vi "Do.vi"(8 "error in (no error)":errorcluster, 10 "Actor in":refnum<class "Actor.lvclass">, 11 "Initiate Acquisition Msg":refnum<class "Initiate Acquisition Msg.lvclass">) -> (0 "error out":errorcluster, 2 "Actor out":refnum<class "Actor.lvclass">)   [LabVIEW 2015, in "CS++Scope.lvlib" / "Initiate Acquisition Msg.lvclass"]
doc: "This VI delivers the message to the actor by calling the appropriate method(s) on the actor."
uses:
  Initiate Acquisition Msg.lvclass
  CS++Scope/CS++Scope.lvclass
  CSPP_Core/Actors/CS++PVMonitor Messages/CS++PVUpdate Msg/CS++PVUpdate Msg.lvclass
  CSPP_Core/Classes/CS++ProcessVariables/ProcessVariable/PV.lvclass
  <vilib>/ActorFramework/Actor/Actor.lvclass
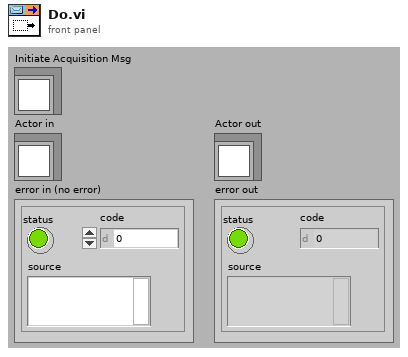
[diagram p1: front panel]
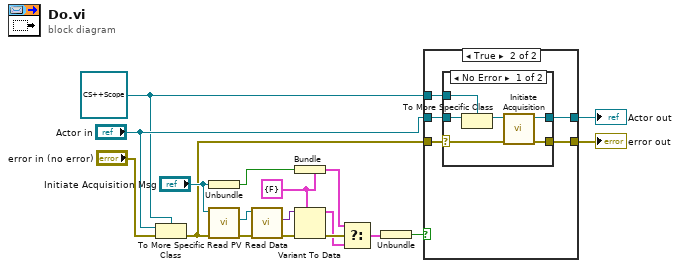
[diagram p0: block diagram]
diagram:
  w4 = cluster{bool} {FALSE} ("Type")
  w14 = refnum<class "CS++Scope.lvclass"> refnum ("Actor in")
  n1 = To More Specific Class(target class=w14, reference="Actor in", error in="error in (no error)") -> (error out=w12:errorcluster)  [unwired: 1 out]
  n2 = Unbundle ("Pre-Unbundler")("Initiate Acquisition Msg") -> (w1:bool)
  n3 = call "Read PV.vi"("error in (no error)"=w12, "CS++PVUpdate Msg in"="Initiate Acquisition Msg") -> ("error out"=w11:errorcluster, "PV"=w3:refnum<class "PV.lvclass">)  [unwired: 7 in, 1 out]
  n4 = call "Read Data.vi"("error in (no error)"=w11, "PV in"=w3) -> ("error out"=w9:errorcluster, "Data"=w10:variant)  [unwired: 7 in, 1 out]
  n5 = Bundle ("Pre-Bundler")(cluster=w4, w1) -> (w7:cluster{bool})
  n6 = Variant To Data(error in=w9, type=w4, Variant=w10) -> (data=w6:cluster{bool}, error out=w8:errorcluster)
  n7 = Select(t=w7, s=w8, f=w6) -> (s? t:f=w5:cluster{bool})
  n8 = Unbundle ("Main-Unbundler")(w5) -> (w2:bool)
  n9 = case "Execute?" shown="True" w2 {
    tunnel: [w19 w25] -> w17
    tunnel: [w20 w24] -> w16
    tunnel: "Actor in" -> [w20 w23]
    tunnel: w14 -> [_ w22]
    tunnel: w12 -> [w19 w21]
    frame False {
    }
    frame True {
      n10 = case shown="No Error" w21 {
        selector: w21 -> [w29 w33]
        tunnel: [w31 w33] -> w25
        tunnel: [w30 w32] -> w24
        tunnel: w23 -> [w28 w32]
        tunnel: w22 -> [w27 _]
        frame No Error {
          n11 = To More Specific Class(target class=w27, reference=w28) -> (specific class reference=w26:refnum<class "CS++Scope.lvclass">)  [unwired: 1 in, 1 out]
          n12 = call "Initiate Acquisition.vi"("error in (no error)"=w29, "CS++Scope"=w26) -> ("error out"=w31:errorcluster, "CS++Scope out"=w30:refnum<class "CS++Scope.lvclass">)  [unwired: 8 in]
        }
        frame Error {
        }
      }
    }
  }
  "error out" <- w17
  "Actor out" <- w16
